vi "Set Distance Callback Threshold.vi"(7 "Callback Option (off)":T1, 8 "error in (no error)":errorcluster, 9 "max":i16, 10 "min":i16, 11 "Distance IR Bricklet in":refnum<class "Distance IR Bricklet.lvclass">) -> (0 "error out":errorcluster, 3 "Distance IR Bricklet out":refnum<class "Distance IR Bricklet.lvclass">)   [LabVIEW 2011, in "Tinkerforge.lvlib" / "Distance IR Bricklet.lvclass"]
doc: "This VI sets the threshold configuration of the distance callback."
uses:
  Distance IR Bricklet.lvclass
  Device/Type Definitions/Callback Option.ctl
  Device/Device.lvclass
  IP Connection/IP Connection.lvclass
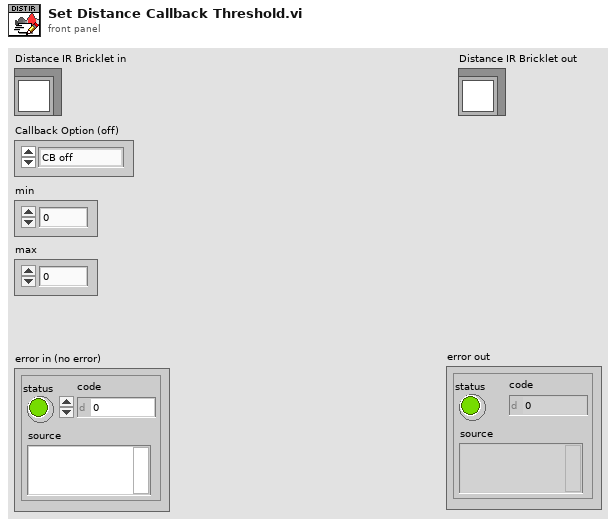
[diagram p1: front panel]
types:
  T1 = typedef "Tinkerforge.lvlib/Device.lvclass/Callback Option.ctl" = enum8{"CB off", "outside range", "inside range", "smaller", "greater"}
  T2 = enum16{"big-endian, network order", "native, host order", "little-endian"}
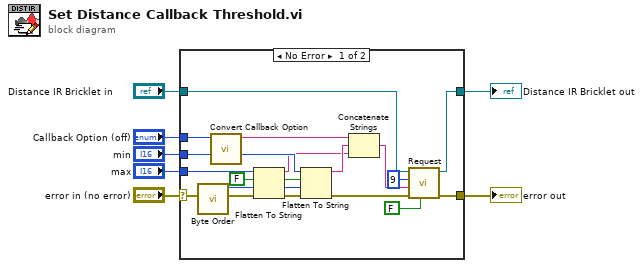
[diagram p0: block diagram]
diagram:
  n1 = case shown="No Error" "error in (no error)" {
    selector: "error in (no error)" -> [w19 w26]
    tunnel: [w20 w26] -> w6
    tunnel: [w23 w25] -> w4
    tunnel: "Distance IR Bricklet in" -> [w24 w25]
    tunnel: "min" -> [w13 _]
    tunnel: "max" -> [w18 _]
    tunnel: "Callback Option (off)" -> [w12 _]
    frame No Error {
      w15 = FALSE ("prepend array or string size? (T)")
      n2 = call "Byte Order.vi"() -> ("byte order (2:little-endian)"=w14:T2)  [unwired: 11 in]
      n3 = call "Convert Callback Option.vi"("Callback Option"=w12) -> ("Callback Option String"=w11:string)  [unwired: 10 in]
      n4 = Flatten To String(anything=w18, prepend array or string size? (T)=w15, byte order (0:big-endian, network order)=w14, error in (no error)=w19) -> (data string=w8:string, error out=w17:errorcluster)  [unwired: 1 out]
      n5 = Flatten To String(anything=w13, prepend array or string size? (T)=w15, byte order (0:big-endian, network order)=w14, error in (no error)=w17) -> (data string=w9:string, error out=w16:errorcluster)  [unwired: 1 out]
      n6 = Concatenate Strings(w11, w9, w8) -> (w10:string)
      n7 = call "Request.vi"("Response"=FALSE, "error in (no error)"=w16, "Data"=w10, "Function ID"=u8 9, "Device in"=w24) -> ("error out"=w20:errorcluster, "Device out"=w23:refnum<class "Distance IR Bricklet.lvclass">)  [unwired: 2 in, 3 out]
    }
    frame Error {
    }
  }
  "error out" <- w6
  "Distance IR Bricklet out" <- w4
